vi "Simple Auto.vi"(10 "Distance to move":dbl) -> ()   [LabVIEW 2013]
uses:
  Robot Global Data.vi
  Device Refrences.vi
  <vilib>/addons/control/pid/pid.llb/PID (DBL).vi
  <vilib>/addons/control/pid/NI_PID_pid.lvlib
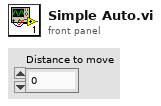
[diagram p1: front panel]
types:
  T1 = cluster{"proportional gain (Kc)":dbl, "integral time (Ti, min)":dbl, "derivative time (Td, min)":dbl}
  T2 = cluster{"Compressor running":bool, "Compressor enabled":bool, "Right Encoder":dbl, "Left Encoder":dbl, "Ultrasonic Sensor":dbl, "Light Sensor":dbl, "Gyro":dbl, "Left Encoder Speed":dbl, "Ball Presence":bool}
  T3 = typedef "WPI_RobotDriveDevRef.ctl" = cluster{"DevStatus":errorcluster, "Motors[]":T4[], "Square Inputs":bool, "Max Output":dbl, "Isochronous":bool}
  T4 = typedef "WPI_MotorControlDeviceRef.ctl" = cluster{"DeviceStatus":errorcluster, "Type":enum16{"PWM", "CAN"}, "PWM":cluster{"Digital Module":T5, "PWM Channel":T6, "DeadBand":T7}, "CAN":cluster{"Device Number":u8, "Control Mode":T8, "Semaphore":T9, "Max Vout":dbl}, "Invert":bool, "TransformRef":T10, "InvTransformRef":T10}
  T5 = typedef "FPGA_TypedefDigitalModule.ctl" = enum16{"Digital Module 1", "Digital Module 2"}
  T6 = typedef "FPGA_DIOPWMChannel.ctl" = enum8{"PWM 1", "PWM 2", "PWM 3", "PWM 4", "PWM 5", "PWM 6", "PWM 7", "PWM 8", "PWM 9", "PWM 10", "Invalid"}
  T7 = typedef "WPI_PWMDeadband.ctl" = cluster{"Name":string, "maxPositivePwm":i32, "minPositivePwm":i32, "centerPwm":i32, "maxNegativePwm":i32, "minNegativePwm":i32, "angularRange":u16}
  T8 = typedef "WPI_CANJaguar_ControlMode.ctl" = enum8{"Percent VBus", "Current", "Speed", "Position", "Voltage"}
  T9 = typedef "Semaphore RefNum" = refnum<k1>
  T10 = typedef "WPI_PWMTransform_ConPane.ctl" = refnum<vi>
  T11 = typedef "WPI_SolenoidValue.ctl" = enum16{"Off", "On", "Forward", "Reverse"}
  T12 = cluster{"Drive Output Values":dbl[], "Shooter Solenoid":T11, "Pickup Solenoid":T11, "Pickup Motor":dbl, "Ejecter Solenoid":T11}
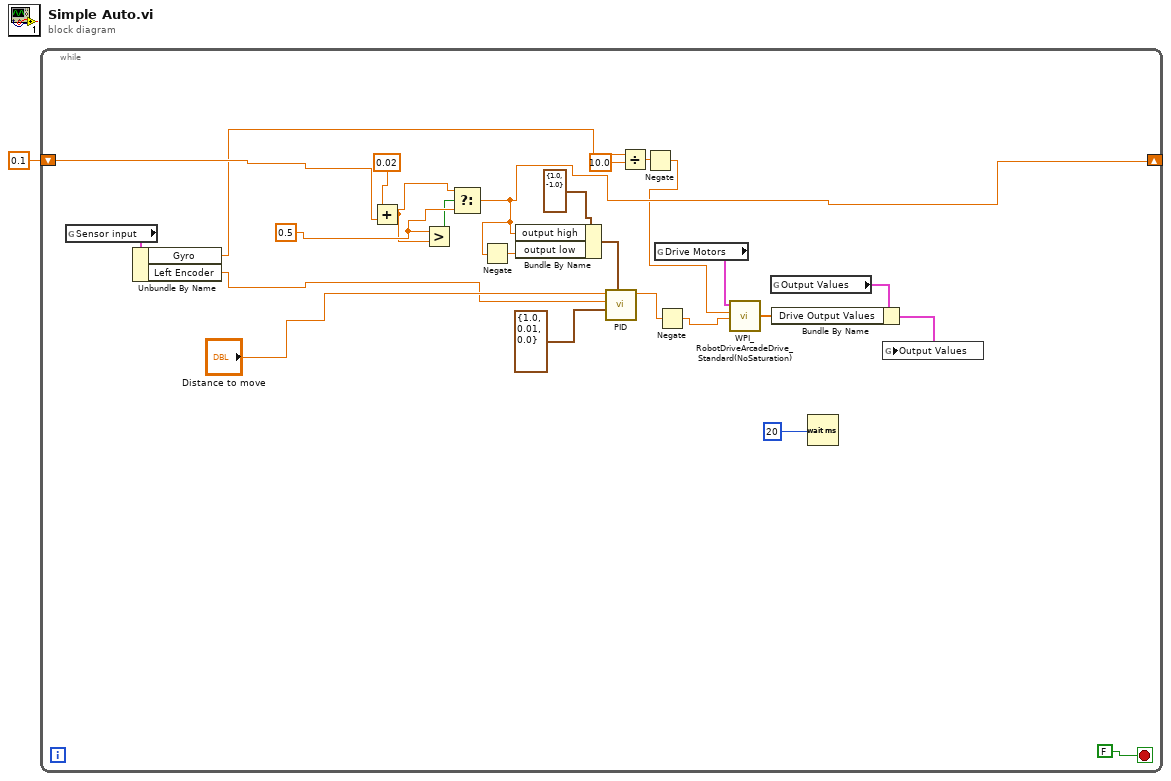
[diagram p0: block diagram]
diagram:
  n1 = while {
    shift-right: [w26] -> _
    shift-left: 0.1 -> [w25]
    stop <- FALSE stop-if-true
    w24 = 0.5
    n2 = global read "Robot Global Data.vi" "Sensor input"() -> (w22:T2)
    n3 = Unbundle By Name(w22) -> ("Gyro"=w20:dbl, "Left Encoder"=w21:dbl)
    n4 = Add(x=0.02, y=w25) -> (x+y=w7:dbl)
    n5 = Greater?(x=w24, y=w7) -> (0:w8:bool)
    n6 = Select(t=w7, s=w8, f=w24) -> (s? t:f=w26:dbl)
    n7 = Negate(x=w26) -> (-x=w9:dbl)
    n8 = Bundle By Name(cluster=cluster{"output high":dbl, "output low":dbl} {"output high"=1.0, "output low"=-1.0} ("output range"), "output high"=w26, "output low"=w9) -> (w12:cluster{"output high":dbl, "output low":dbl})
    n9 = call-poly <vilib>:"PID.vi"("output range"=w12, "PID gains"=T1 {"proportional gain (Kc)"=1.0, "integral time (Ti, min)"=0.01, "derivative time (Td, min)"=0.0}, "process variable"=w21, "setpoint"="Distance to move") -> ("output"=w14:dbl)  [unwired: 6 in, 1 out]
    n10 = Divide(x=w20, y=10.0) -> (x/y=w4:dbl)
    n11 = Negate(x=w4) -> (-x=w3:dbl)
    n12 = global read "Device Refrences.vi" "Drive Motors"() -> (w17:T3)
    n13 = Negate(x=w14) -> (-x=w13:dbl)
    n14 = call <vilib>:"WPI_RobotDriveArcadeDrive_Standard(NoSaturation).vi"("Y axis value"=w13, "X axis value"=w3, "RobotDriveDevRef"=w17) -> ("Motor Values"=w18:dbl[])  [unwired: 1 in, 7 out]
    n15 = global read "Robot Global Data.vi" "Output Values"() -> (w16:T12)
    n16 = Bundle By Name(cluster=w16, "Drive Output Values"=w18) -> (w15:T12)
    n17 = Wait (ms)(milliseconds to wait=20) -> ()  [unwired: 1 out]
    n18 = global write "Robot Global Data.vi" "Output Values"(w15) -> ()
  }
